vi "ProcessHeaderData.vi"(8 "error in":errorcluster, 11 "Binary string":string) -> (0 "error out":errorcluster, 1 "Packet length":u16, 2 "Packet type":u16, 3 "Binary string without header":string, 5 "Sync Id":u32)   [LabVIEW 2020, in "SmartEyeProDriver.lvclass"]
uses:
  SmartEyeProDriver.lvclass
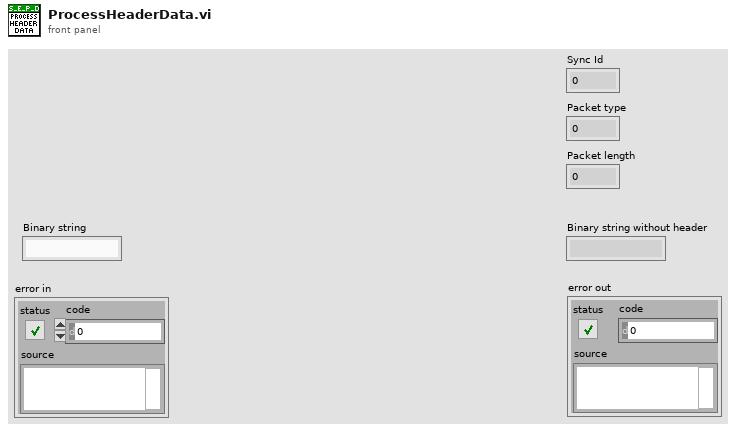
[diagram p1: front panel]
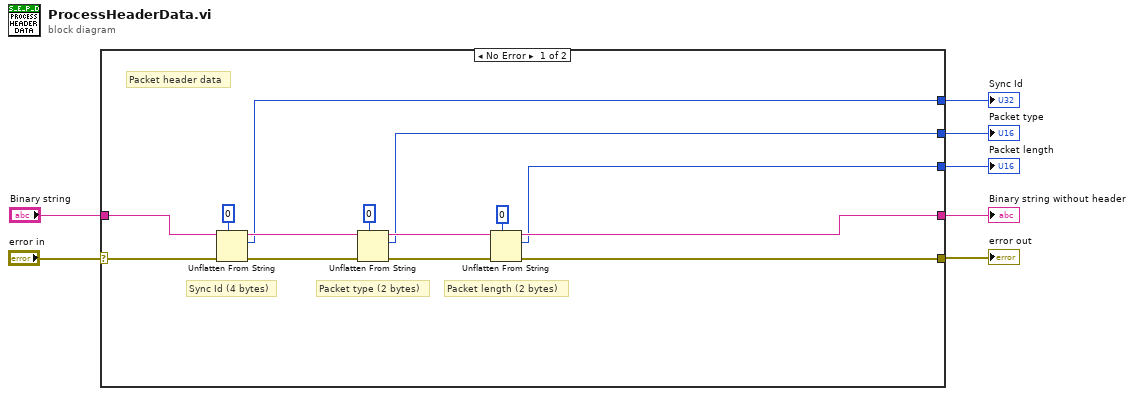
[diagram p0: block diagram]
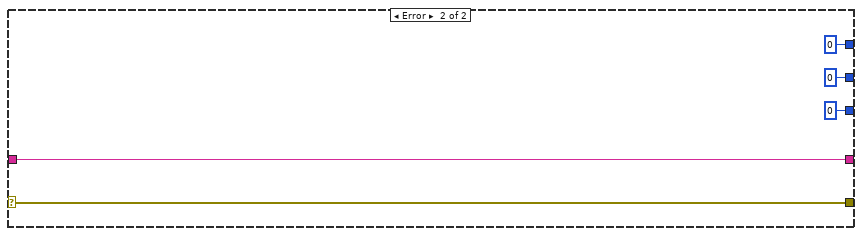
[diagram p2: hidden frame]
diagram:
  n1 = case shown="No Error" "error in" {
    selector: "error in" -> [w14 w26]
    tunnel: [w11 w26] -> w4
    tunnel: "Binary string" -> [w13 w25]
    tunnel: [w12 w25] -> w5
    tunnel: [w10 u16 0] -> w3
    tunnel: [w9 u16 0] -> w2
    tunnel: [w8 u32 0] -> w1
    frame No Error {
      # "Packet header data"
      # "Packet type (2 bytes)"
      # "Packet length (2 bytes)"
      # "Sync Id (4 bytes)"
      n2 = Unflatten From String(type=u32 0, binary string=w13, error in (no error)=w14) -> (rest of the binary string=w16:string, value=w8:u32, error out=w17:errorcluster)  [unwired: 2 in]
      n3 = Unflatten From String(type=u16 0, binary string=w16, error in (no error)=w17) -> (rest of the binary string=w19:string, value=w9:u16, error out=w18:errorcluster)  [unwired: 2 in]
      n4 = Unflatten From String(type=u16 0, binary string=w19, error in (no error)=w18) -> (rest of the binary string=w12:string, value=w10:u16, error out=w11:errorcluster)  [unwired: 2 in]
    }
    frame Error {
    }
  }
  "error out" <- w4
  "Binary string without header" <- w5
  "Packet length" <- w3
  "Packet type" <- w2
  "Sync Id" <- w1
